vi "build output string - strobe.vi"(1 "Array of \"period-units\"":i32[](array[numeric])) -> (0 "output string":string)   [LabVIEW 2009]
doc: "Takes an input array x of \"period units\" and builds and output string accordingly. The output string has:\nx(0) number of 0s, then\nx(1) number of 1s, then\nx(2) number of 0s, then\nx(3) number of 1s, and so on."
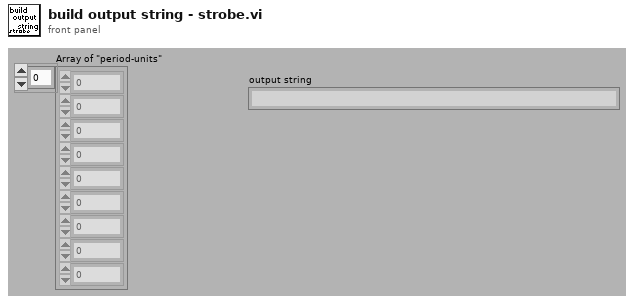
[diagram p1: front panel]
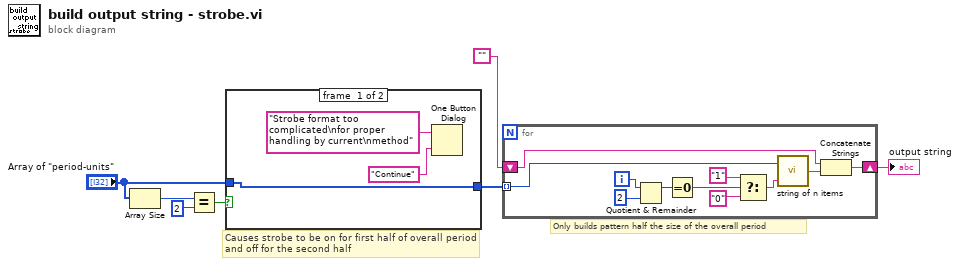
[diagram p0: block diagram]
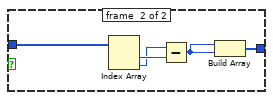
[diagram p2: hidden frame]
diagram:
  # "Causes strobe to be on for first half of overall period\nand off for the second half"
  # "Only builds pattern half the size of the overall period"
  n1 = Array Size(array="Array of \"period-units\"") -> (size(s)=w5:i32)
  n2 = Equal?(x=w5, y=2) -> (x = y?=w3:bool)
  n3 = case shown="True" w3 {
    tunnel: "Array of \"period-units\"" -> [w10 w15]
    tunnel: [w10 w13] -> w1
    frame #0 {
      n4 = One Button Dialog(message="Strobe format too complicated\nfor proper handling by current\nmethod", button name ("OK")="Continue") -> ()  [unwired: 1 out]
    }
    frame #1 {
      n5 = Index Array(array=w15) -> (element #1=w14:i32, element #2=w12:i32)  [unwired: 2 in]
      n6 = Subtract(x=w12, y=w14) -> (x-y=w11:i32)
      n7 = Build Array(w11, w11) -> (w13:i32[])
    }
  }
  n8 = for {
    tunnel: w1 -> [w19] mode=indexing
    shift-right: [w17] -> w6
    shift-left: "" -> [w18]
    i -> [w23]
    n9 = Quotient & Remainder(x=w23, y=2) -> (x-y*floor(x/y)=w25:i32)  [unwired: 1 out]
    n10 = Equal To 0?(x=w25) -> (x = 0?=w24:bool)
    n11 = Select(t="1", s=w24, f="0") -> (s? t:f=w22:string)
    n12 = call "string of n items.vi"("string"=w22, "Numeric"=w19) -> ("String"=w16:string)
    n13 = Concatenate Strings(w18, w16) -> (w17:string)
  }
  "output string" <- w6
